vi "DrawOverlayImage.vi"(0 "reference":refnum<class "AbstractNode.lvclass">, 1 "graphics":refnum<class "Graphics.lvclass">, 5 "error in (no error)":errorcluster) -> (14 "reference out":refnum<class "AbstractNode.lvclass">, 15 "HotSpots":T1[](array[typedef]) {"HotSpot"."y" format="%.2f"; "HotSpot"."x" format="%.2f"}, 19 "error out":errorcluster)   [LabVIEW 2020, in "AbstractNode.lvclass"]
uses:
  <resource>/Framework/Providers/Open_GDS/UML/AbstractNode_class/AbstractNode.lvclass
  <resource>/Framework/Providers/Open_GDS/UML/Graphics_class/Graphics.lvclass
  <resource>/Framework/Providers/Open_GDS/UML/UMLEditor/UMLEditor_HotSpotData.ctl
  <resource>/Framework/Providers/Open_GDS/UML/General/Point/Point Point2D.ctl
  <resource>/Framework/Providers/Open_GDS/UML/UMLEditor/UMLEditor_HotSpotType.ctl
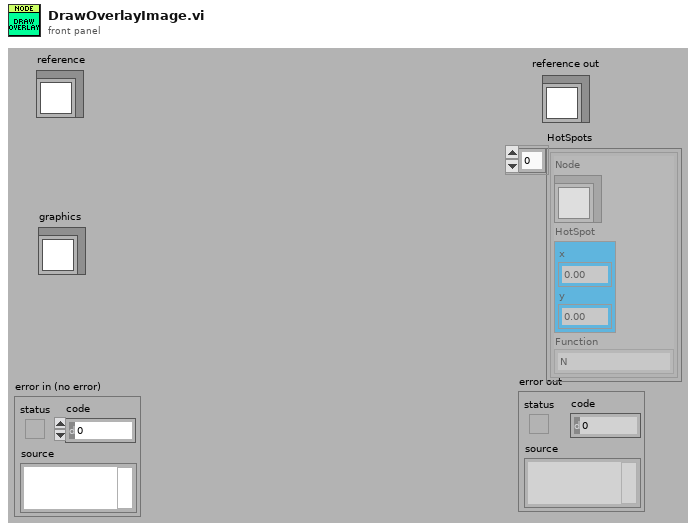
[diagram p1: front panel]
types:
  T1 = typedef "UMLEditor_HotSpotData.ctl" = cluster{"Node":refnum<class "AbstractNode.lvclass">, "HotSpot":T2, "Function":T3}
  T2 = typedef "Point Point2D.ctl" = cluster{"x":dbl, "y":dbl}
  T3 = typedef "UMLEditor_HotSpotType.ctl" = enum16{"N", "NE", "E", "SE", "S", "SW", "W", "NW", "Expand", "Collaps"}
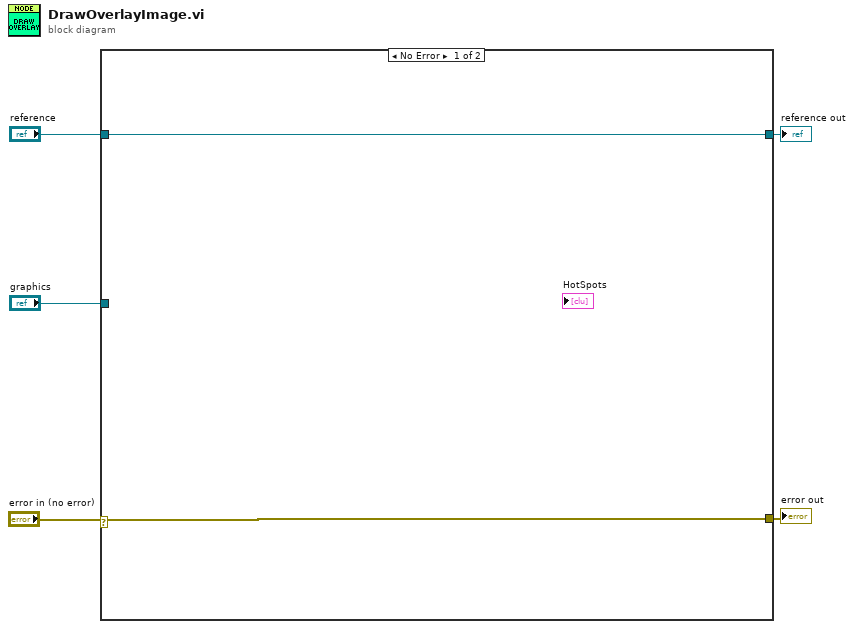
[diagram p0: block diagram]
diagram:
  n1 = case shown="No Error" "error in (no error)" {
    selector: "error in (no error)" -> [w7 w8]
    tunnel: "reference" -> [w6 w9]
    tunnel: [w7 w8] -> w4
    tunnel: [w6 w9] -> w3
    tunnel: "graphics" -> [_ _]
    frame No Error {
    }
    frame Error {
    }
  }
  "reference out" <- w3
  "error out" <- w4
